vi "MoveRight.vi"(0 "Grids In":i32[][](array[numeric])) -> (1 "Grids Out":i32[][](array[numeric]), 2 "Score":i32, 3 "Moved?":bool)   [LabVIEW 2018]
doc: "Move grids right."
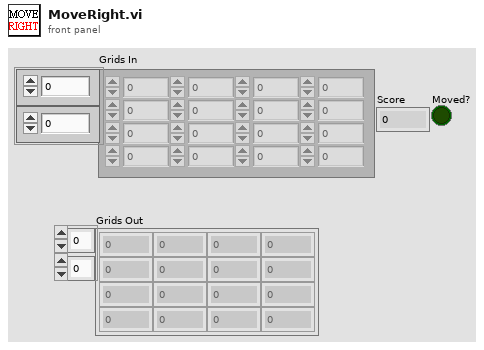
[diagram p1: front panel]
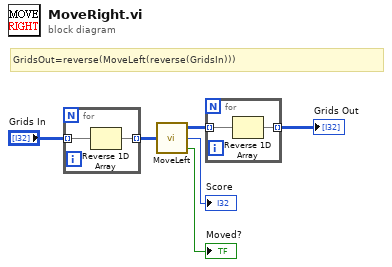
[diagram p0: block diagram]
diagram:
  # "GridsOut=reverse(MoveLeft(reverse(GridsIn)))"
  n1 = for {
    tunnel: "Grids In" -> [w8] mode=indexing
    tunnel: [w7] -> w5 mode=indexing
    n2 = Reverse 1D Array(array=w8) -> (reversed array=w7:i32[])
  }
  n3 = call "MoveLeft.vi"("Grids In"=w5) -> ("Grid Out"=w4:i32[][], "Score"=→"Score":i32, "Moved?"=→"Moved?":bool)
  n4 = for {
    tunnel: w4 -> [w10] mode=indexing
    tunnel: [w9] -> w3 mode=indexing
    n5 = Reverse 1D Array(array=w10) -> (reversed array=w9:i32[])
  }
  "Grids Out" <- w3
